vi "Get Network Devices.vi"(4 "Network Adapters (F)":bool, 6 "Local Subnet Only (T)":bool caption="Local Subnet Only (F)", 8 "Error in":errorcluster, 9 "Device Class String":string[](array[string]), 10 "Device Class":T4, 11 "SysCfg Device in":refnum<class "SysCfg Device.lvclass">) -> (0 "Error out":errorcluster, 1 "Devices Skipped":T1[](array[typedef]) {"Product ID" format="%.0x"; "Primary Network Adapter"."IP Address Request Mode" items=["Static"=1, "DHCP/Link Local"=2, "Link-Local Only"=4, "DHCP Only"=8]; "Primary Network Adapter"."Adapter Type" items=["Ethernet"=1, "WLAN"=2]; "Primary Network Adapter"."Adapter Mode" items=["Disabled"=1, "TCP/IP Ethernet"=2, "Deterministic"=4, "EtherCAT"=8, "TCP/IP WLAN Connect"=32, "TCP/IP WLAN Create"=64]; "Secondary Network Adapters"."IP Address Request Mode" items=["Static"=1, "DHCP/Link Local"=2, "Link-Local Only"=4, "DHCP Only"=8]; "Secondary Network Adapters"."Adapter Type" items=["Disabled"=1, "TCP/IP Ethernet"=2, "Deterministic"=4, "EtherCAT"=8, "TCP/IP WLAN Connect"=32, "TCP/IP WLAN Create"=64]; "Secondary Network Adapters"."Adapter Mode" items=["Disabled"=1, "TCP/IP Ethernet"=2, "Deterministic"=4, "EtherCAT"=8, "TCP/IP WLAN Connect"=32, "TCP/IP WLAN Create"=64]}, 2 "Devices Found":T1[](array[typedef]) {"Product ID" format="%.0x"; "Primary Network Adapter"."IP Address Request Mode" items=["Static"=1, "DHCP/Link Local"=2, "Link-Local Only"=4, "DHCP Only"=8]; "Primary Network Adapter"."Adapter Type" items=["Ethernet"=1, "WLAN"=2]; "Primary Network Adapter"."Adapter Mode" items=["Disabled"=1, "TCP/IP Ethernet"=2, "Deterministic"=4, "EtherCAT"=8, "TCP/IP WLAN Connect"=32, "TCP/IP WLAN Create"=64]; "Secondary Network Adapters"."IP Address Request Mode" items=["Static"=1, "DHCP/Link Local"=2, "Link-Local Only"=4, "DHCP Only"=8]; "Secondary Network Adapters"."Adapter Type" items=["Disabled"=1, "TCP/IP Ethernet"=2, "Deterministic"=4, "EtherCAT"=8, "TCP/IP WLAN Connect"=32, "TCP/IP WLAN Create"=64]; "Secondary Network Adapters"."Adapter Mode" items=["Disabled"=1, "TCP/IP Ethernet"=2, "Deterministic"=4, "EtherCAT"=8, "TCP/IP WLAN Connect"=32, "TCP/IP WLAN Create"=64]}, 3 "SysCfg Device out":refnum<class "SysCfg Device.lvclass">)   [LabVIEW 2015, in "SMI.lvlib" / "SysCfg Device.lvclass"]
uses:
  SysCfg Device/SysCfg Device.lvclass
  Controller/Controls/NetworkDevice.ctl
  Controller/Controls/DeviceInformation.ctl
  Controller/Controls/NetworkAdapterSettings.ctl
  Device/Controls/DeviceClassSelection.ctl
  SysCfg Device/SysCfg Device.lvclass/SysCfg Device.ctl
  Controller/Controller.lvclass
  Device/Device.lvclass
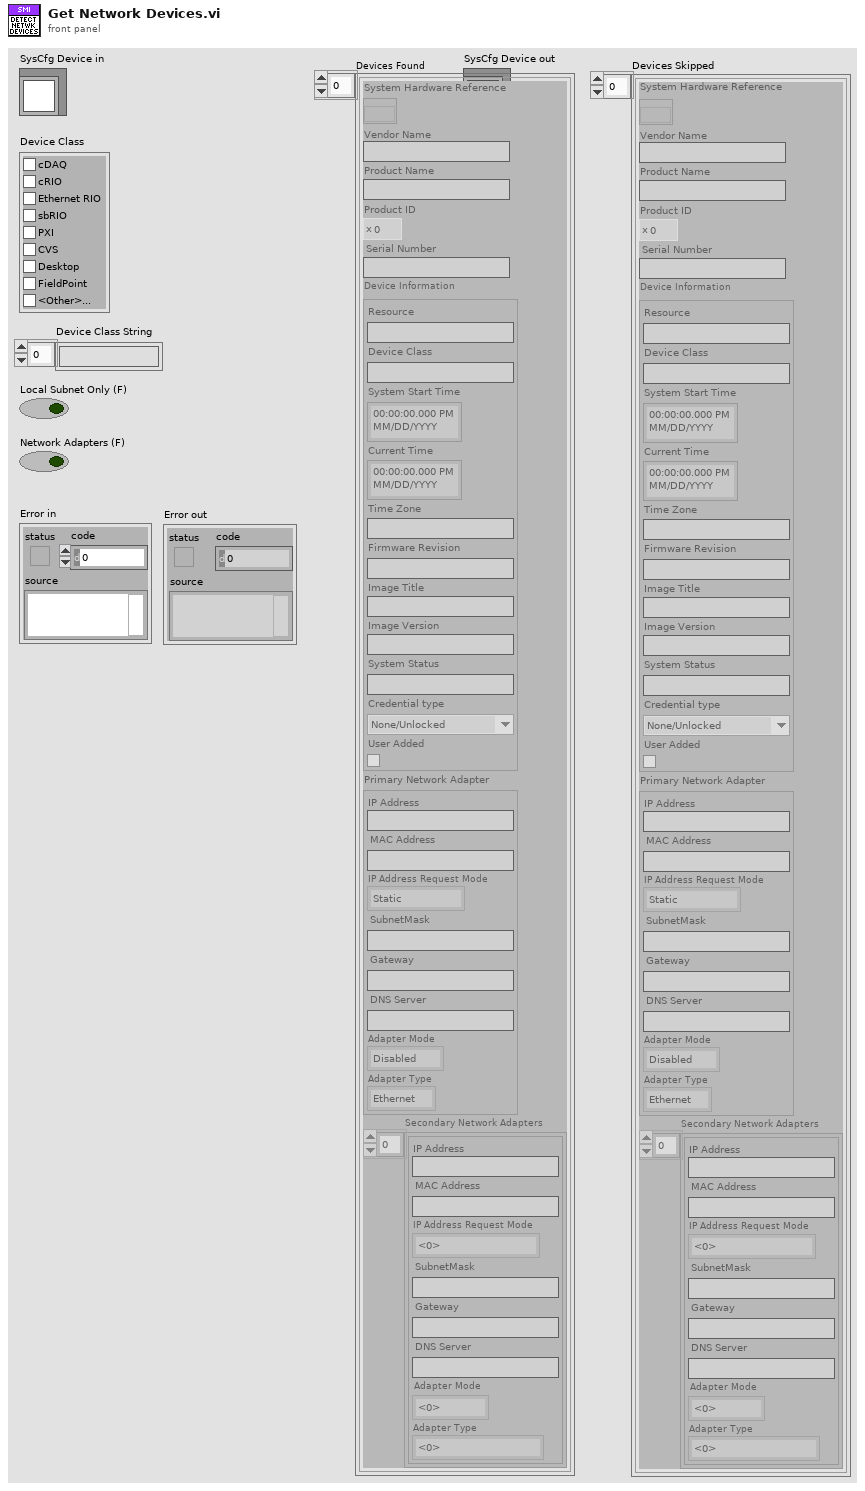
[diagram p1: front panel]
types:
  T1 = typedef "SMI.lvlib/Controller.lvclass/NetworkDevice.ctl" = cluster{"System Hardware Reference":refnum<k20>, "Vendor Name":string, "Product Name":string, "Product ID":u32, "Serial Number":string, "Device Information":T2, "Primary Network Adapter":T3, "Secondary Network Adapters":T3[]}
  T2 = typedef "SMI.lvlib/Controller.lvclass/DeviceInformation.ctl" = cluster{"Resource":string, "Device Class":string, "System Start Time":timestamp, "Current Time":timestamp, "Time Zone":string, "Firmware Revision":string, "Image Title":string, "Image Version":string, "System Status":string, "Credential type":enum16{"None/Unlocked", "FTP Password", "NIAuth Credentials"}, "User Added":bool}
  T3 = typedef "SMI.lvlib/Controller.lvclass/NetworkAdapterSettings.ctl" = cluster{"IP Address":string, "MAC Address":string, "IP Address Request Mode":u32, "SubnetMask":string, "Gateway":string, "DNS Server":string, "Adapter Mode":u32, "Adapter Type":u32}
  T4 = typedef "SMI.lvlib/Device.lvclass/DeviceClassSelection.ctl" = cluster{"cDAQ":bool, "cRIO":bool, "Ethernet RIO":bool, "sbRIO":bool, "PXI":bool, "CVS":bool, "Desktop":bool, "FieldPoint":bool, "<Other>...":bool}
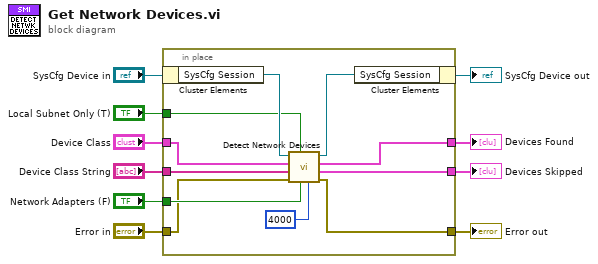
[diagram p0: block diagram]
diagram:
  n1 = in-place {
    in-place-border: "Local Subnet Only (T)" -> [w19]
    in-place-border: "Network Adapters (F)" -> [w17]
    in-place-border: "Error in" -> [w16]
    in-place-border: [w15] -> w9
    in-place-border: "Device Class String" -> [w14]
    in-place-border: "Device Class" -> [w13]
    in-place-border: [w12] -> w6
    in-place-border: [w11] -> w1
    n2 = in-place-cluster #1("SysCfg Device in") -> ("SysCfg Session"=w21:refnum<k21>)
    n3 = call "Detect Network Devices.vi"("Remote Timeout"=u32 4000 ("Timeout (4000 ms)"), "Network Adapters"=w17, "Local Subnet Only"=w19, "Error in"=w16, "Device Class String"=w14, "Device Class"=w13, "Session in (localhost)"=w21) -> ("Error out"=w15:errorcluster, "Devices Skipped"=w11:T1[], "Devices Found"=w12:T1[], "Session out"=w20:refnum<k21>)  [unwired: 1 in]
    n4 = in-place-cluster #1("SysCfg Session"=w20) -> (→"SysCfg Device out":refnum<class "SysCfg Device.lvclass">)
  }
  "Error out" <- w9
  "Devices Found" <- w6
  "Devices Skipped" <- w1
